vi "makeDecisions.vi"(8 "error in (no error)":errorcluster, 10 "model":refnum<class "Model.lvclass">, 11 "RampingUpPressureSTState in":refnum<class "RampingUpPressureSTState.lvclass">) -> (0 "error out":errorcluster, 2 "model 2":refnum<class "Model.lvclass">, 3 "RampingUpPressureSTState out":refnum<class "RampingUpPressureSTState.lvclass">)   [LabVIEW 2015, in "RampingUpPressureSTState.lvclass"]
uses:
  RampingUpPressureSTState.lvclass
  Model/Model/Model.lvclass
  Typedefs/StateSelector.ctl
  TestingStiffnessState/TestingStiffnessState.lvclass
  Typedefs/M1M3SSSTypedefs.lvlib
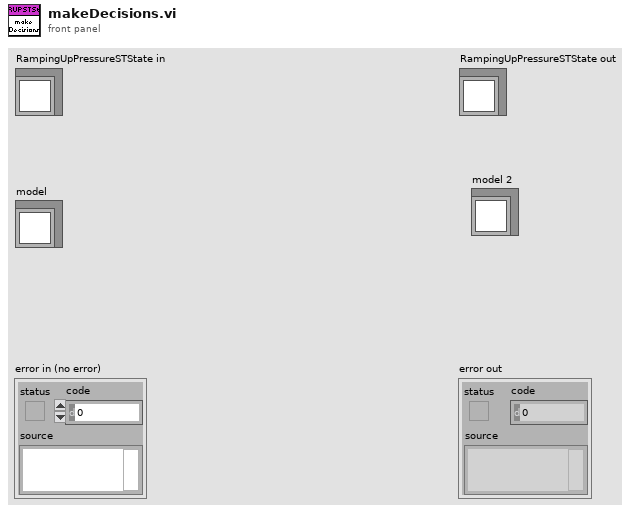
[diagram p1: front panel]
types:
  T1 = typedef "M1M3SSSTypedefs.lvlib/StateSelector.ctl" = enum16{"FaultState", "OffState", "RampingUpPressurePState", "RampingUpPressureSTState", "StandbyState", "StoppedState", "WaitingForSettledPState", "WaitingForSettledSTState"}
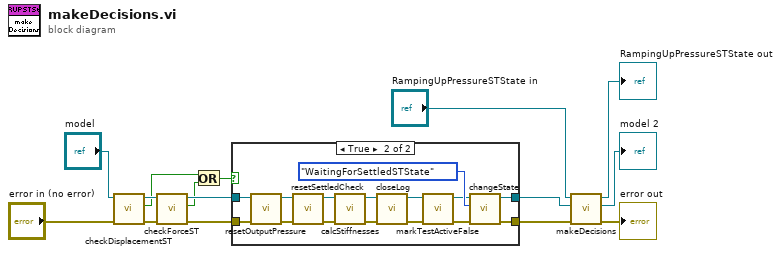
[diagram p0: block diagram]
diagram:
  n1 = call "checkDisplacementST.vi"("error in (no error)"="error in (no error)", "Model in"="model") -> ("error out"=w5:errorcluster, "reachedDisplacementTriggerIsTrue"=w3:bool, "Model out"=w7:refnum<class "Model.lvclass">)  [unwired: 7 in]
  n2 = call "checkForceST.vi"("error in (no error)"=w5, "Model in"=w7) -> ("error out"=w4:errorcluster, "reachedForceTriggerIsTrue"=w2:bool, "Model out"=w6:refnum<class "Model.lvclass">)  [unwired: 7 in]
  n3 = Or(x=w3, y=w2) -> (x .or. y?=w1:bool)
  n4 = case shown="True" w1 {
    tunnel: w6 -> [w17 w30]
    tunnel: w4 -> [w16 w29]
    tunnel: [w16 w32] -> w9
    tunnel: [w17 w31] -> w10
    frame False {
    }
    frame True {
      n5 = call "resetOutputPressure.vi"("error in (no error)"=w29, "Model in"=w30) -> ("error out"=w26:errorcluster, "Model out"=w27:refnum<class "Model.lvclass">)  [unwired: 8 in]
      n6 = call "resetSettledCheck.vi"("error in (no error)"=w26, "Model in"=w27) -> ("error out"=w24:errorcluster, "Model out"=w25:refnum<class "Model.lvclass">)  [unwired: 7 in, 1 out]
      n7 = call "calcStiffnesses.vi"("error in (no error)"=w24, "Model in"=w25) -> ("error out"=w22:errorcluster, "Model out"=w23:refnum<class "Model.lvclass">)  [unwired: 8 in]
      n8 = call "closeLog.vi"("error in (no error)"=w22, "Model in"=w23) -> ("error out"=w19:errorcluster, "Model out"=w21:refnum<class "Model.lvclass">)  [unwired: 8 in]
      n9 = call "markTestActiveFalse.vi"("error in (no error)"=w19, "Model in"=w21) -> ("error out"=w18:errorcluster, "Model out"=w20:refnum<class "Model.lvclass">)  [unwired: 8 in]
      n10 = call "changeState.vi"("error in (no error)"=w18, "State:"=StateSelector."WaitingForSettledSTState", "Model in"=w20) -> ("error out"=w32:errorcluster, "Model out"=w31:refnum<class "Model.lvclass">)  [unwired: 7 in]
    }
  }
  n11 = call-parent "makeDecisions.vi"("error in (no error)"=w9, "model"=w10, "EnabledState in"="RampingUpPressureSTState in") -> ("error out"=→"error out":errorcluster, "model 2"=→"model 2":refnum<class "Model.lvclass">, "EnabledState out"=→"RampingUpPressureSTState out":refnum<class "RampingUpPressureSTState.lvclass">)  [unwired: 6 in]
